vi "GlobalDoubles.vi"(2 "Write Value":dbl format="%.2f", 3 "Element":i32, 4 "Operation":i32 min=0 max=1, 5 "Number of elements":i32=30) -> (0 "Double Array Out":dbl[](array[numeric]) format="%.2f", 1 "Read Value":dbl format="%.2f")   [LabVIEW 2015]
doc: "Handle Double Globals Style II.\nThe globals are maintained in a\nshift register, as an array of doubles.\nTherefore, it is mandatory to initialize each element\nof the array with the first invocation wiring\nthe number of elements to be contained in\nthe array. The elements will be initialized to 0.0\n\nINPUTS:\n Number of elements: Use only on first call\n to initialize the array\n Operation: 1 = WRITE; 0 = READ\n Element: Element of the array to write or read\n Write Value: Double value to store\nOUTPUTS:\n Read Value: Double value retrieved\n Double Array Out: The entire array of doubles."
panel:
  # "1 = WRITE"
  # "0 = READ"
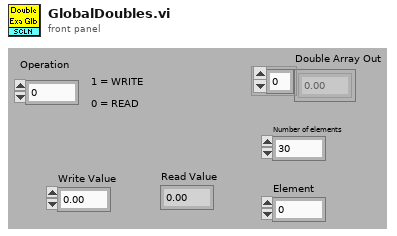
[diagram p1: front panel]
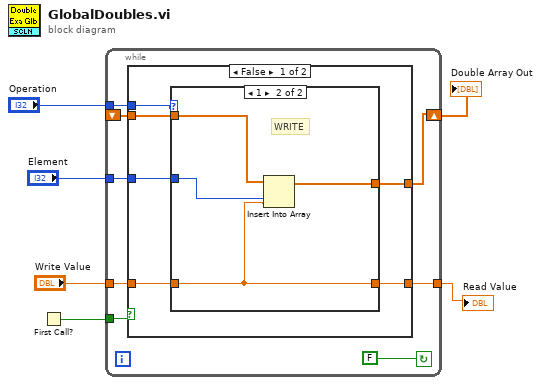
[diagram p0: block diagram]
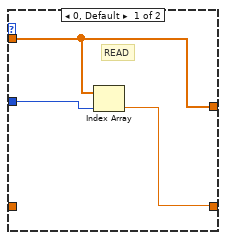
[diagram p2: hidden frame]
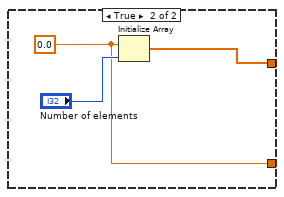
[diagram p3: hidden frame]
diagram:
  n1 = First Call?() -> (First Call?: T/F=w1:bool)
  n2 = while {
    shift-right: [w9] -> w3
    shift-left: _ -> [w10]
    tunnel: "Operation" -> [w13]
    tunnel: "Element" -> [w12]
    tunnel: "Write Value" -> [w11]
    tunnel: [w8] -> w2
    tunnel: w1 -> [w7]
    stop <- FALSE continue-if-true
    n3 = case shown="False" w7 {
      tunnel: w13 -> [w20 _]
      tunnel: w12 -> [w19 _]
      tunnel: w11 -> [w18 _]
      tunnel: w10 -> [w17 _]
      tunnel: [w16 w29] -> w9
      tunnel: [w15 w28] -> w8
      frame False {
        n4 = case shown="1" w20 {
          tunnel: w19 -> [w21 w27]
          tunnel: w18 -> [_ w24]
          tunnel: w17 -> [w23 w26]
          tunnel: [w23 w25] -> w16
          tunnel: [w22 w24] -> w15
          frame 0, Default {
            # "READ"
            n5 = Index Array(array=w23, index=w21) -> (element=w22:dbl)
          }
          frame 1 {
            # "WRITE"
            n6 = Insert Into Array(array=w26, index=w27, new element=w24) -> (w25:dbl[])
          }
        }
      }
      frame True {
        w28 = 0.0
        n7 = Initialize Array(w28, "Number of elements") -> (w29:dbl[])
      }
    }
  }
  "Double Array Out" <- w3
  "Read Value" <- w2
